vi "dash safety data FG.vi"(2 "Mechanism":enum16{"Drive Train"}(ring), 5 "Menu":T1) -> ()   [LabVIEW 2013]
uses:
  typedefs/fg_getset.ctl
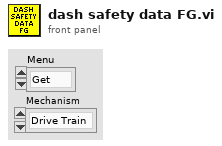
[diagram p1: front panel]
types:
  T1 = typedef "fg_getset.ctl" = enum16{"Get", "Set"}
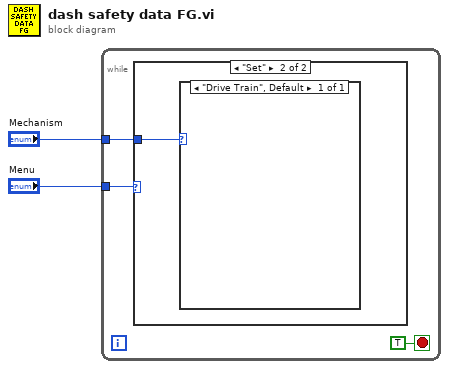
[diagram p0: block diagram]
diagram:
  n1 = while {
    tunnel: "Menu" -> [w4]
    tunnel: "Mechanism" -> [w3]
    stop <- TRUE stop-if-true
    n2 = case shown="\"Set\"" w4 {
      tunnel: w3 -> [_ w6]
      frame "Get", Default {
      }
      frame "Set" {
        n3 = case shown="\"Drive Train\", Default" w6 {
          frame "Drive Train", Default {
          }
        }
      }
    }
  }
